vi "Open_id.vi"(4 "error in (no error)":errorcluster, 6 "Device id string":string) -> (0 "error out":errorcluster, 3 "Device handle":u32 format="%x")   [LabVIEW 2014, in "MBUG-2820.lvlib"]
doc: "Opens a device specified by the id string (MBUG-2820-XXXXXX).\nReturns a device handle which must be passed to all functions accessing the device."
uses:
  <instrlib>/MBUG-2820/MBUG-2820.lvlib
  <instrlib>/MBUG-2820/mbugdll.dll
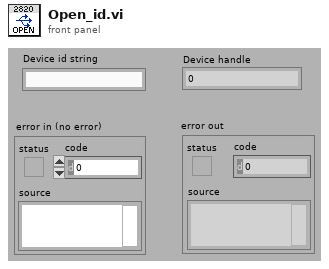
[diagram p1: front panel]
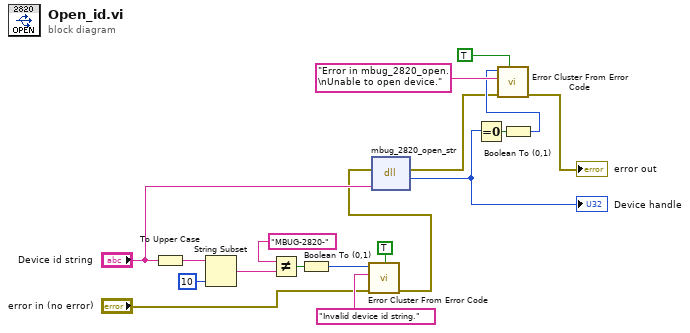
[diagram p0: block diagram]
diagram:
  n1 = To Upper Case(1:"Device id string") -> (0:w11:string)
  n2 = String Subset(string=w11, length (rest)=10 ("length (rest)")) -> (substring=w2:string)  [unwired: 1 in]
  n3 = Not Equal?(x="MBUG-2820-" ("y"), y=w2) -> (x != y?=w6:bool)
  n4 = Boolean To (0,1)(Boolean=w6) -> (0, 1=w7:i16)
  n5 = call <vilib>:"Error Cluster From Error Code.vi"("show call chain? (False)"=TRUE, "error in (no error)"="error in (no error)", "error message (\"\")"="Invalid device id string.", "error code (0)"=w7) -> ("error out"=w4:errorcluster)  [unwired: 5 in]
  n6 = dll-call lib="C:/Programme/National Instruments/LabVIEW 2014/instr.lib/MBUG-2820/mbugdll.dll" fn="mbug_2820_open_str"(error in=w4, "serial_num"="Device id string") -> (error out=w13:errorcluster, "dev_handle"=w17:u64)  [unwired: 3 in, 1 out]
  "Device handle" <- w17
  n7 = Equal To 0?(x=w17) -> (x = 0?=w15:bool)
  n8 = Boolean To (0,1)(Boolean=w15) -> (0, 1=w14:i16)
  n9 = call <vilib>:"Error Cluster From Error Code.vi"("show call chain? (False)"=TRUE, "error in (no error)"=w13, "error message (\"\")"="Error in mbug_2820_open.\nUnable to open device.", "error code (0)"=w14) -> ("error out"=→"error out":errorcluster)  [unwired: 5 in]
